vi "PicoScope4000aExampleRapidBlockBulkOverlapped.vi"() -> ()   [LabVIEW 2010]
doc: "This example demonstrates how to use the PicoScope Labview library to collect data using rapid block mode, retrieving the data values in bulk."
uses:
  shared/PicoBuffers.ctl
  PicoScope4000aLib/PicoScope4000aAnalogChannelSettings.ctl
  shared/Segment Range.ctl
  shared/Buffer and Transfer Settings.ctl
  shared/Acquisition Settings.ctl
  shared/nSegments.ctl
panel:
  in  "Channel B Settings":T1={"Enabled"=FALSE, "Coupling"=1, "Range"=6, "Analogue Offset"=0.0, "Bandwidth Limit"=0} {"Bandwidth Limit" items=["Full", "20kHz", "100kHz", "1MHz"]; "Range" items=["10 mV", "20 mV", "50 mV", "100 mV", "200 mV", "500 mV", "1 V", "2 V", "5 V", "10 V", "20 V", "50 V ", "100 V"]; "Coupling" items=["AC", "DC"]}
  in  "roundFaster":bool
  in  "timeIntervalRequested":dbl format="%#6_6p"
  in  "Write to TDMS":bool
  in  "Resolution":u32(ring)=1 items=["8-bit", "12-bit", "14-bit"]
  out "Unit Info":T2
  in  "Trigger Settings":T3={"Trigger Enabled"=FALSE, "Trigger Source"=enum."Channel A", "Trigger Threshold (Volts/Probe units)"=0.0, "Trigger Direction"=2, "Trigger Delay (samples)"=0, "Auto Trigger Time (ms)"=1000} {"Trigger Direction" items=["Rising"=2, "Falling"=3]}
  out "overflow":i16[](array[numeric]) format="%08b"
  in  "Channel A Settings":T1={"Enabled"=TRUE, "Coupling"=1, "Range"=6, "Analogue Offset"=0.0, "Bandwidth Limit"=0} {"Bandwidth Limit" items=["Full", "20kHz", "100kHz", "1MHz"]; "Range" items=["10 mV", "20 mV", "50 mV", "100 mV", "200 mV", "500 mV", "1 V", "2 V", "5 V", "10 V", "20 V", "50 V ", "100 V"]; "Coupling" items=["AC", "DC"]}
  out "USB 3.0 device on non-USB 3.0 Port":bool
  out "USB Powered":bool=TRUE
  in  "Stop Display":bool
  out "Capture Complete":bool
  in  "Run":bool
  in  "Display Buffer Index":i32
  in  "Segment Range":T4={"fromSegmentIndex"=0, "toSegmentIndex"=9} {"toSegmentIndex" format="%.4p"; "fromSegmentIndex" format="%.4p"}
  in  "nSegments":T5=10 format="%#.4p"
  out "error out":errorcluster
  in  "Data file":path=path "PicoScope4000aExampleRapidBlock ChA Data"
  in  "Buffer and Transfer Settings":T6={"startIndex"=0, "Samples"=5000000, "Down Sample Ratio"=1, "Down-Sample Mode"=0} {"Down-Sample Mode" items=["RAW none"=2147483648, "None"=0, "Aggregate"=1, "Decimate"=2, "Average"=4]; "Down Sample Ratio" step=1; "Samples" format="%_6p"}
  in  "Acquisition Settings":T7={"preTriggerSamples"=0, "postTriggerSamples"=5000000, "timebase"=0} {"postTriggerSamples" format="%_6p"; "preTriggerSamples" format="%_6p"}
  out "Properties Panel":T8={"Sample Frequency"=41666668.0, "Sample Rate"=2.4000000209412065e-08, "Max Samples Available"=26843008, "Number of Samples"=0, "Total Capture Time (sec) "=0.0, "Max Total Capture Time Available (sec)"=0.6442322134971619} {"Max Total Capture Time Available (sec)" format="%.3p"; "Sample Frequency" format="%.6p"; "Sample Rate" format="%.3p"; "Max Samples Available" format="%_6p"; "Total Capture Time (sec)" format="%.3p"}
  in  "stop":bool
  out "Analog Channels":cluster{i32, dbl, "Data":dbl[]}[](graph)
  in  "Serial Number":string
  in  "Use Serial Number":bool
  in  "error in (no error)":errorcluster
  # "Number of\nSegments to Capture"
  # "Bit 0 = ChA"
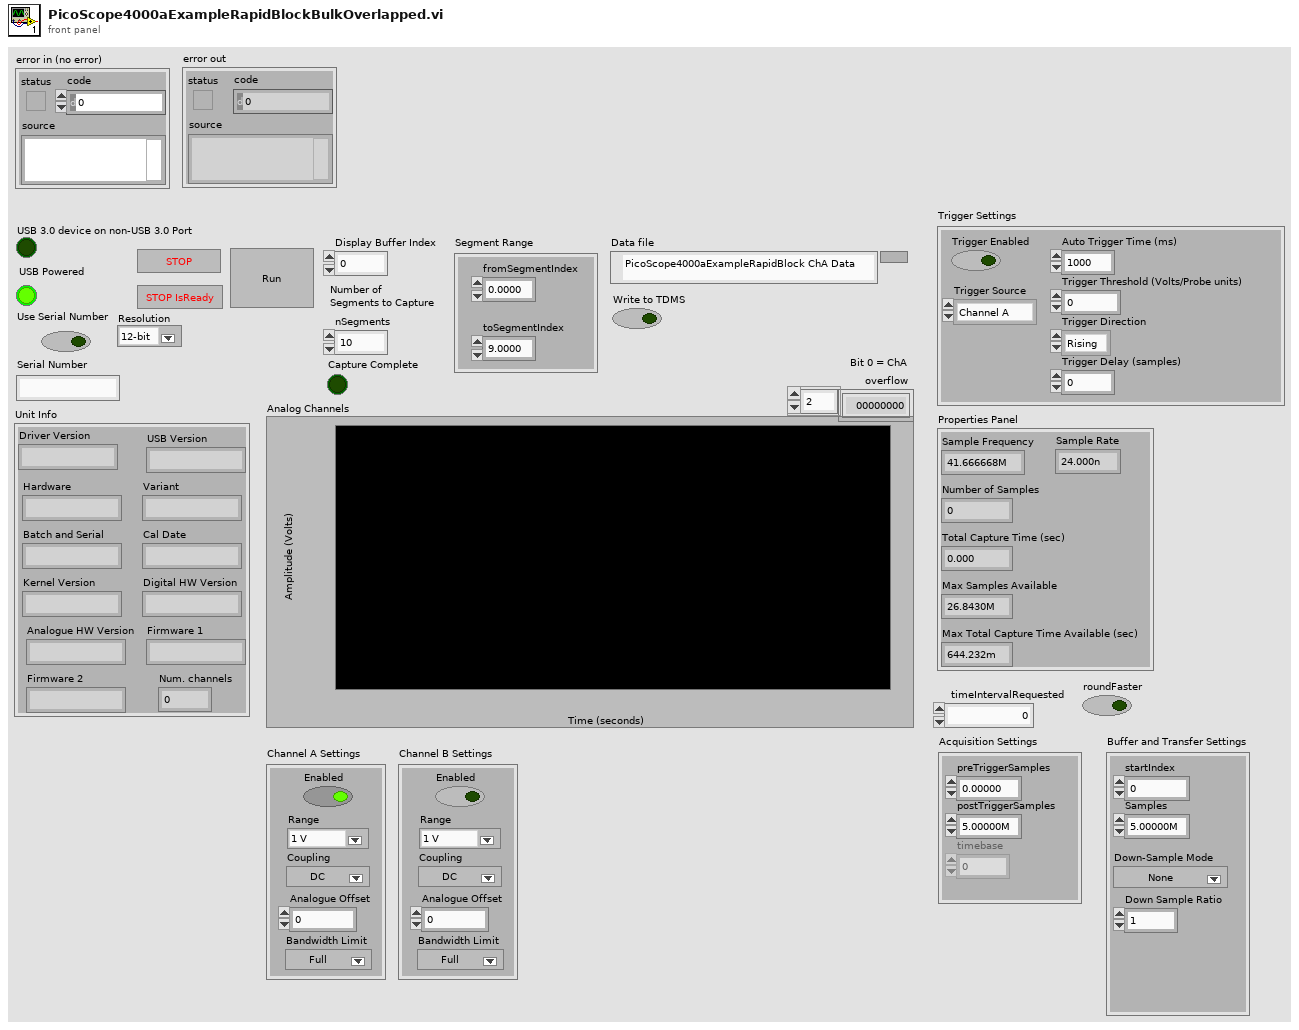
[diagram p1: front panel]
types:
  T1 = typedef "PicoScope4000aAnalogChannelSettings.ctl" = cluster{"Enabled":bool, "Coupling":i16, "Range":u32, "Analogue Offset":sgl, "Bandwidth Limit":u32}
  T2 = cluster{"Driver Version":string, "USB Version":string, "Hardware":string, "Variant":string, "Batch and Serial":string, "Cal Date":string, "Kernel Version":string, "Digital HW Version":string, "Analogue HW Version":string, "Firmware 1":string, "Firmware 2":string, "Num. channels":i16}
  T3 = cluster{"Trigger Enabled":bool, "Trigger Source":enum16{"Channel A", "Channel B", "Channel C", "Channel D", "Channel E", "Channel F", "Channel G", "Channel H"}, "Trigger Threshold (Volts/Probe units)":dbl, "Trigger Direction":u16, "Trigger Delay (samples)":u32, "Auto Trigger Time (ms)":i16}
  T4 = typedef "Segment Range.ctl" = cluster{"fromSegmentIndex":u64, "toSegmentIndex":u64}
  T5 = typedef "nSegments.ctl" = u64
  T6 = typedef "Buffer and Transfer Settings.ctl" = cluster{"startIndex":u64, "Samples":u64, "Down Sample Ratio":u64, "Down-Sample Mode":u32}
  T7 = typedef "Acquisition Settings.ctl" = cluster{"preTriggerSamples":u64, "postTriggerSamples":u64, "timebase":u32}
  T8 = cluster{"Sample Frequency":dbl, "Sample Rate":dbl, "Max Samples Available":u64, "Number of Samples":u64, "Total Capture Time (sec) ":dbl, "Max Total Capture Time Available (sec)":dbl}
  T9 = typedef "PicoBuffers.ctl" = cluster{"Max Buffer Pointers":u64[][][], "Min Buffer Pointers":u64[][][], "StreamingDataInfo":cluster{"Channel":u32, "Down-Sample Mode":u32, "PICO_DATA_TYPE":enum32{"PICO_INT8_T", "PICO_INT16_T", "PICO_INT32_T", "PICO_UINT32_T", "PICO_INT64_T", ""}, "Samples":i32, "bufferIndex":u64, "startIndex":i32, "overflow":i16}[][]}
  T10 = enum16{"open", "open or create", "create or replace", "create", "open (read-only)"}
  T11 = cluster{"Channel A Buffer":i16[], "Channel B Buffer":i16[], "Channel C Buffer":i16[], "Channel D Buffer":i16[], "Channel E Buffer":i16[], "Channel F Buffer":i16[], "Channel G Buffer":i16[], "Channel H Buffer":i16[], "Port 0 Buffer":i16[], "Port 1 Buffer":i16[]}[]
  T12 = cluster{"Channel A Buffer":i16[], "Channel B Buffer":i16[], "Channel C Buffer":i16[], "Channel D Buffer":i16[], "Channel E Buffer":i16[], "Channel F Buffer":i16[], "Channel G Buffer":i16[], "Channel H Buffer":i16[], "Port 0 Buffer":i16[], "Port 1 Buffer":i16[]}
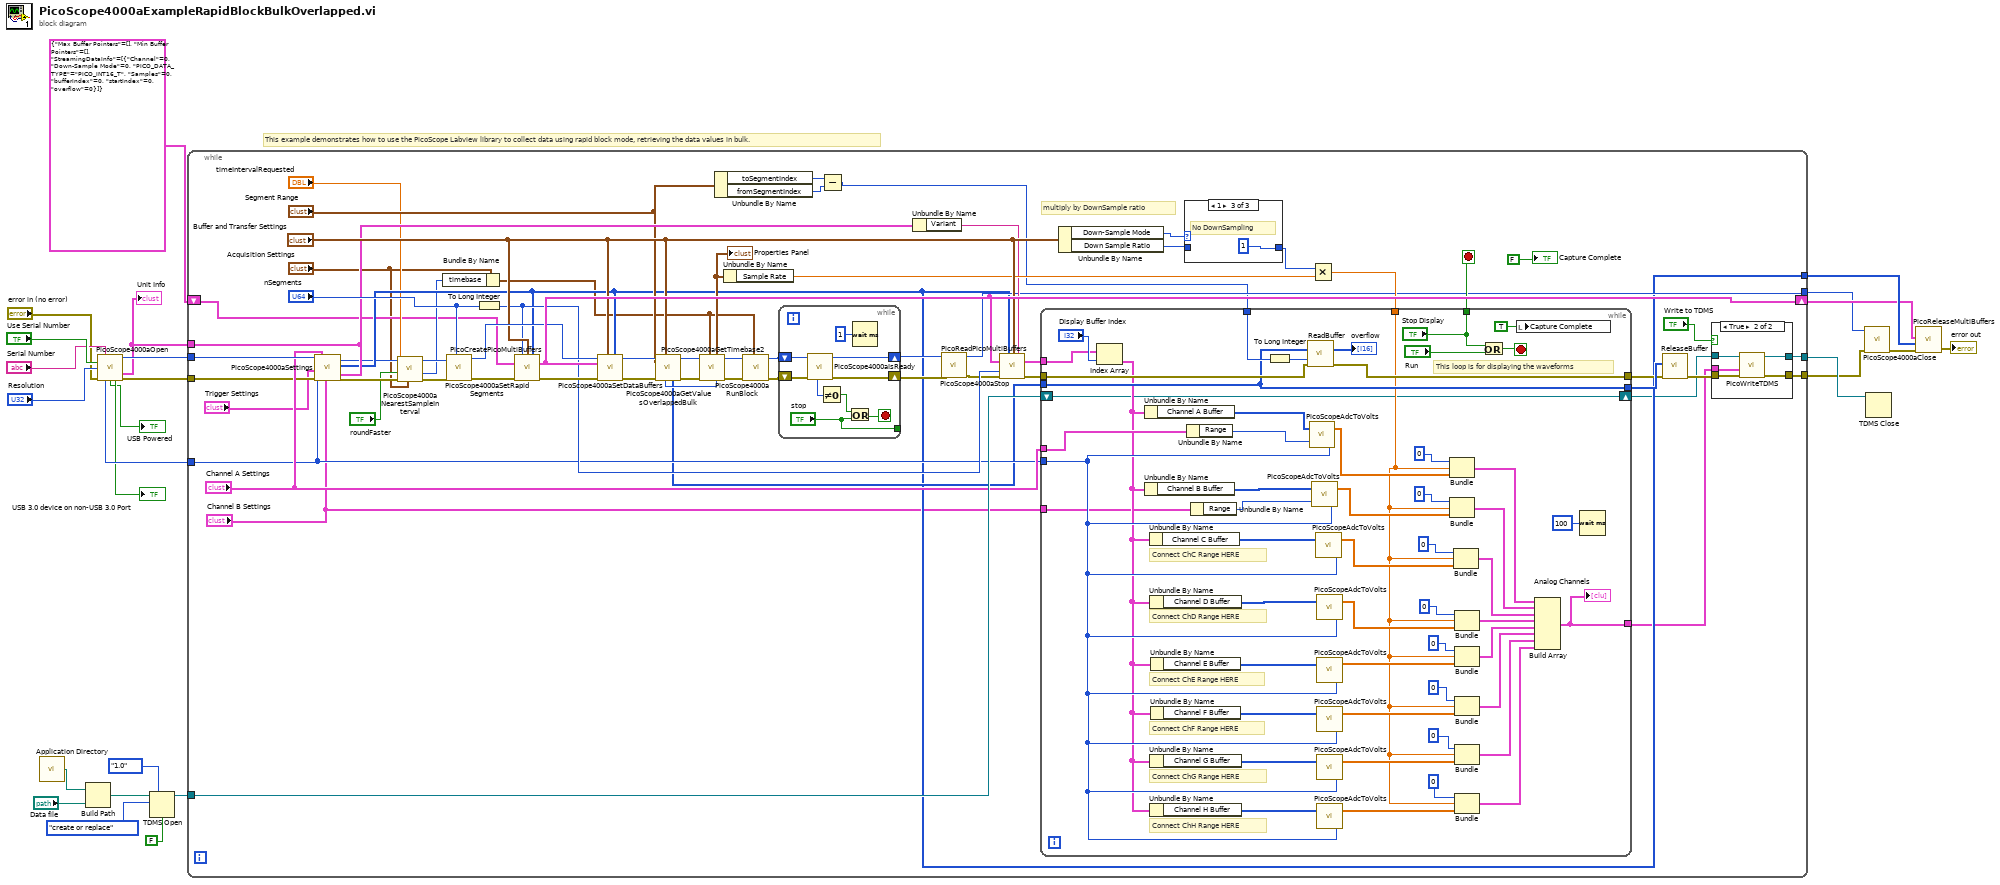
[diagram p0: block diagram]
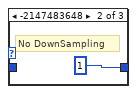
[diagram p4: hidden frame]
diagram:
  # "This example demonstrates how to use the PicoScope Labview library to collect data using rapid block mode, retrieving the data values in bulk."
  n1 = call <vilib>:"Application Directory.vi"() -> ("Application Directory"=w17:path)
  n2 = Build Path(base path=w17, name or relative path="Data file") -> (appended path=w18:path)
  n3 = call "PicoScope4000aOpen.vi"("Serial Number"="Serial Number", "Use Serial Number"="Use Serial Number", "Resolution"="Resolution", "error in (no error)"="error in (no error)") -> ("handle"=w12:i16, "Unit Info"=w3:T2, "Max ADC value"=w13:i16, "USB powered"=→"USB Powered":bool, "USB 3.0 on non-USB 3.0 port"=→"USB 3.0 device on non-USB 3.0 Port":bool, "error out"=w4:errorcluster)  [unwired: 4 in, 2 out]
  "Unit Info" <- w3
  n4 = TDMS Open(6:FALSE ("disable buffering? (T)"), 7:enum16{"1.0", "2.0"}."1.0" ("file format version (2.0)"), 10:T10."create or replace" ("operation (0:open)"), 11:w18) -> (3:w15:refnum<k34>)  [unwired: 2 in, 1 out]
  n5 = while {
    tunnel: w13 -> [w63]
    tunnel: [w54] -> w23
    tunnel: [w43] -> w25
    tunnel: [w40] -> w16
    tunnel: w15 -> [w86]
    tunnel: w3 -> [w60]
    tunnel: w12 -> [w66]
    tunnel: w4 -> [w45]
    tunnel: [w37] -> w2
    shift-right: [w87] -> w24
    shift-left: T9 {"Max Buffer Pointers"=[], "Min Buffer Pointers"=[], "StreamingDataInfo"=[[{"Channel"=0, "Down-Sample Mode"=0, "PICO_DATA_TYPE"=enum."PICO_INT16_T", "Samples"=0, "bufferIndex"=0, "startIndex"=0, "overflow"=0}]]} ("Data Pointers") -> [w27]
    stop <- w71 stop-if-true
    # "multiply by DownSample ratio"
    n6 = call "PicoScope4000aSettings.vi"("handle in"=w66, "Trigger Settings"="Trigger Settings", "Max ADC value"=w63, "error in"=w45, "Channel A Settings"="Channel A Settings", "Channel B Settings"="Channel B Settings", "Unit Info"=w60) -> ("handle out"=w33:i16, "Enabled array"=w43:i16[], "error out"=w36:errorcluster)  [unwired: 10 in]
    n7 = call "PicoScope4000aNearestSampleInterval.vi"("Acquisition Settings"="Acquisition Settings", "error in (no error)"=w36, "roundFaster"="roundFaster", "timeIntervalRequested"="timeIntervalRequested", "handle in"=w33) -> ("error out"=w35:errorcluster, "timebase"=w31:u32, "handle out"=w34:i16)  [unwired: 3 in, 1 out]
    n8 = Bundle By Name(cluster="Acquisition Settings", "timebase"=w31) -> (w32:T7)
    n9 = call "PicoScope4000aSetRapidSegments.vi"("nSegments"="nSegments", "error in (no error)"=w35, "handle in"=w34) -> ("error out"=w85:errorcluster, "handle out"=w84:i16)  [unwired: 6 in, 1 out]
    n10 = To Long Integer(number="nSegments") -> (32bit integer=w64:i32)
    n11 = call "PicoCreatePicoMultiBuffers.vi"("Number of Buffers"=w64, "Buffer and Transfer Settings"="Buffer and Transfer Settings", "enabled array"=w43, "Data Pointers In"=w27, "error in (no error)"=w85) -> ("Data Pointers"=w87:T9, "error out"=w88:errorcluster)  [unwired: 9 in]
    n12 = call "PicoScope4000aSetDataBuffers.vi"("enabled array"=w43, "Buffer and Transfer Settings"="Buffer and Transfer Settings", "error in (no error)"=w88, "Data Pointers In"=w87, "handle in"=w84) -> ("error out"=w83:errorcluster, "handle out"=w82:i16)  [unwired: 5 in]
    n13 = call "PicoScope4000aGetValuesOverlappedBulk.vi"("Segment Range"="Segment Range", "Buffer and Transfer Settings"="Buffer and Transfer Settings", "error in (no error)"=w83, "handle in"=w82) -> ("error out"=w58:errorcluster, "handle out"=w59:i16, "Pointer to Overflow"=w48:u64[], "noOfSamples"=w53:u64)  [unwired: 4 in]
    n14 = call "PicoScope4000aGetTimebase2.vi"("Number of Samples"=w53, "Acquisition Settings"=w32, "error in (no error)"=w58, "handle in"=w59) -> ("error out"=w56:errorcluster, "handle out"=w57:i16, "Properties Panel"=w77:T8)  [unwired: 5 in]
    "Properties Panel" <- w77
    n15 = Unbundle By Name("Segment Range") -> ("toSegmentIndex"=w52:u64, "fromSegmentIndex"=w51:u64)
    n16 = Unbundle By Name(w77) -> ("Sample Rate"=w62:dbl)
    n17 = call "PicoScope4000aRunBlock.vi"("Acquisition Settings"=w32, "error in (no error)"=w56, "handle in"=w57) -> ("error out"=w74:errorcluster, "handle out"=w73:i16)  [unwired: 5 in, 2 out]
    n18 = while {
      shift-right: [w157] -> w68
      shift-left: w74 -> [w158]
      shift-right: [w156] -> w67
      shift-left: w73 -> [w155]
      tunnel: ["stop"] -> _
      stop <- w152 stop-if-true
      n19 = call "PicoScope4000aIsReady.vi"("error in (no error)"=w158, "handle in"=w155) -> ("error out"=w157:errorcluster, "handle out"=w156:i16, "ready"=w154:i16)  [unwired: 7 in]
      n20 = Not Equal To 0?(x=w154) -> (x != 0?=w153:bool)
      n21 = Or(x=w153, y="stop") -> (x .or. y?=w152:bool)
      n22 = Wait (ms)(milliseconds to wait=u32 1) -> ()  [unwired: 1 out]
    }
    n23 = Subtract(x=w52, y=w51) -> (x-y=w49:u64)
    n24 = Unbundle By Name(w60) -> ("Variant"=w61:string)
    n25 = call "PicoScope4000aStop.vi"("error in (no error)"=w68, "handle in"=w67) -> ("error out"=w55:errorcluster, "handle out"=w54:i16)  [unwired: 8 in]
    n26 = call "PicoReadPicoMultiBuffers.vi"("enabled array"=w43, "Buffer and Transfer Settings"="Buffer and Transfer Settings", "Variant"=w61, "Data Pointers"=w87, "No of Buffers"=w64, "error in (no error)"=w55) -> ("MultiBuffers (Max or non-aggregated)"=w80:T11, "error out"=w72:errorcluster)  [unwired: 7 in, 1 out]
    n27 = Unbundle By Name("Buffer and Transfer Settings") -> ("Down-Sample Mode"=w78:u32, "Down Sample Ratio"=w79:u64)
    n28 = case shown="1" w78 {
      tunnel: [w159 u64 1 ("Down Sample Ratio") u64 1 ("Down Sample Ratio")] -> w75
      tunnel: w79 -> [w159 _ _]
      frame Default {
      }
      frame -2147483648 {
        # "No DownSampling"
      }
      frame 1 {
        # "No DownSampling"
      }
    }
    n29 = Multiply(x=w75, y=w62) -> (x*y=w76:dbl)
    n30 = while {
      tunnel: w63 -> [w106]
      tunnel: "Channel A Settings" -> [w149]
      tunnel: w80 -> [w133]
      tunnel: w76 -> [w103]
      shift-right: [w99] -> w39
      shift-left: w86 -> [w99]
      tunnel: [w123] -> w46
      tunnel: w72 -> [w122]
      tunnel: ["Stop Display"] -> w71
      tunnel: w49 -> [w121]
      tunnel: w48 -> [w119]
      tunnel: [w119] -> w47
      tunnel: [w98] -> w38
      tunnel: "Channel B Settings" -> [w96]
      stop <- w136 stop-if-true
      # "Connect ChE Range HERE"
      # "Connect ChH Range HERE"
      # "Connect ChG Range HERE"
      # "Connect ChF Range HERE"
      # "This loop is for displaying the waveforms"
      # "Connect ChD Range HERE"
      # "Connect ChC Range HERE"
      n31 = Index Array(array=w133, index="Display Buffer Index") -> (element=w105:T12)
      n32 = Unbundle By Name(w105) -> ("Channel A Buffer"=w140:i16[])
      n33 = Unbundle By Name(w105) -> ("Channel B Buffer"=w145:i16[])
      n34 = Unbundle By Name(w105) -> ("Channel C Buffer"=w131:i16[])
      n35 = Unbundle By Name(w105) -> ("Channel D Buffer"=w127:i16[])
      n36 = Unbundle By Name(w105) -> ("Channel G Buffer"=w117:i16[])
      n37 = Unbundle By Name(w105) -> ("Channel H Buffer"=w116:i16[])
      n38 = Unbundle By Name(w105) -> ("Channel E Buffer"=w115:i16[])
      n39 = Unbundle By Name(w105) -> ("Channel F Buffer"=w118:i16[])
      n40 = Unbundle By Name(w149) -> ("Range"=w147:u32)
      n41 = Unbundle By Name(w96) -> ("Range"=w97:u32)
      n42 = To Long Integer(number=w121) -> (32bit integer=w120:i32)
      n43 = call "ReadBuffer.vi"("Pointer and BufferSize"=w119, "Buffer size"=w120, "error in (no error)"=w122) -> ("Output Array"=→"overflow":i16[], "error out"=w123:errorcluster)  [unwired: 11 in]
      n44 = call "PicoScopeAdcToVolts.vi"("Max_adc"=w106, "Range Index"=w147, "Data"=w140) -> ("Data"=w141:dbl[])
      n45 = call "PicoScopeAdcToVolts.vi"("Max_adc"=w106, "Range Index"=w97, "Data"=w145) -> ("Data"=w144:dbl[])
      n46 = call "PicoScopeAdcToVolts.vi"("Max_adc"=w106, "Data"=w131) -> ("Data"=w130:dbl[])  [unwired: 1 in]
      n47 = call "PicoScopeAdcToVolts.vi"("Max_adc"=w106, "Data"=w127) -> ("Data"=w126:dbl[])  [unwired: 1 in]
      n48 = call "PicoScopeAdcToVolts.vi"("Max_adc"=w106, "Data"=w115) -> ("Data"=w114:dbl[])  [unwired: 1 in]
      n49 = call "PicoScopeAdcToVolts.vi"("Max_adc"=w106, "Data"=w118) -> ("Data"=w109:dbl[])  [unwired: 1 in]
      n50 = call "PicoScopeAdcToVolts.vi"("Max_adc"=w106, "Data"=w117) -> ("Data"=w108:dbl[])  [unwired: 1 in]
      n51 = call "PicoScopeAdcToVolts.vi"("Max_adc"=w106, "Data"=w116) -> ("Data"=w107:dbl[])  [unwired: 1 in]
      n52 = Bundle(0, w103, "Data"=w141) -> (w143:cluster{i32, dbl, "Data":dbl[]})  [unwired: 1 in]
      n53 = Bundle(0, w103, "Data"=w144) -> (w142:cluster{i32, dbl, "Data":dbl[]})  [unwired: 1 in]
      n54 = Bundle(0, w103, "Data"=w130) -> (w129:cluster{i32, dbl, "Data":dbl[]})  [unwired: 1 in]
      n55 = Bundle(0, w103, "Data"=w126) -> (w125:cluster{i32, dbl, "Data":dbl[]})  [unwired: 1 in]
      n56 = Bundle(0, w103, "Data"=w114) -> (w104:cluster{i32, dbl, "Data":dbl[]})  [unwired: 1 in]
      n57 = Bundle(0, w103, "Data"=w109) -> (w102:cluster{i32, dbl, "Data":dbl[]})  [unwired: 1 in]
      n58 = Bundle(0, w103, "Data"=w108) -> (w101:cluster{i32, dbl, "Data":dbl[]})  [unwired: 1 in]
      n59 = Bundle(0, w103, "Data"=w107) -> (w100:cluster{i32, dbl, "Data":dbl[]})  [unwired: 1 in]
      n60 = Or(x="Stop Display", y="Run") -> (x .or. y?=w136:bool)
      n61 = local write "Capture Complete"(TRUE ("Capture Complete")) -> ()
      n62 = Build Array(w143, w142, w129, w125, w104, w102, w101, w100) -> (w98:cluster{i32, dbl, "Data":dbl[]}[])
      "Analog Channels" <- w98
      n63 = Wait (ms)(milliseconds to wait=u32 100) -> ()  [unwired: 1 out]
    }
    n64 = call "ReleaseBuffer.vi"("error in (no error)"=w46, "Pointer and BufferSize"=w47) -> ("error out"=w41:errorcluster)  [unwired: 9 in]
    n65 = case shown="True" "Write to TDMS" {
      tunnel: w38 -> [_ w95]
      tunnel: w39 -> [w89 w94]
      tunnel: w41 -> [w90 w93]
      tunnel: [w90 w92] -> w37
      tunnel: [w89 w91] -> w40
      frame False {
      }
      frame True {
        n66 = call "PicoWriteTDMS.vi"("error in (no error)"=w93, "Analog Channels"=w95, "Refnum in"=w94) -> ("error out"=w92:errorcluster, "Refnum out"=w91:refnum<k34>)  [unwired: 7 in]
      }
    }
    "Capture Complete" <- FALSE ("Capture Complete")
  }
  n67 = call "PicoScope4000aClose.vi"("error in (no error)"=w2, "handle in"=w23) -> ("error out"=w6:errorcluster)  [unwired: 7 in, 1 out]
  n68 = TDMS Close(11:w16) -> ()  [unwired: 1 in, 2 out]
  n69 = call "PicoReleaseMultiBuffers.vi"("error in (no error)"=w6, "Enabled array"=w25, "Data Pointers"=w24) -> ("error out"=→"error out":errorcluster)  [unwired: 7 in, 1 out]
